vi "GOOP_WirePenTranslator.vi"(1 "WireConfigurationIn":T2, 3 "WirePensIn":T1(array[cluster])) -> (15 "WirePensOut":T1(array[cluster]), 17 "WireConfigurationOut":T2)   [LabVIEW 2020]
uses:
  <resource>/Framework/Providers/Open_GDS/SubVIs/GOOP_WireConfigurationType.ctl
  <resource>/Framework/Providers/Open_GDS/SubVIs/GOOP_WirePattern.ctl
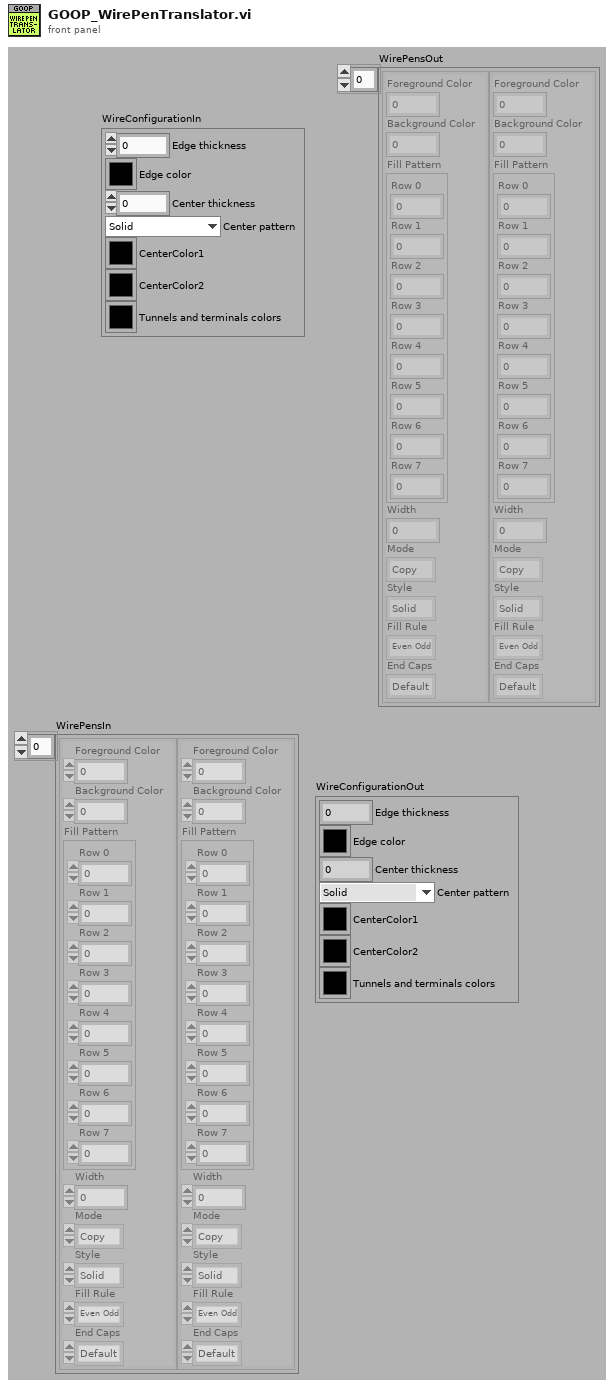
[diagram p1: front panel]
types:
  T1 = cluster{"Foreground Color":u32, "Background Color":u32, "Fill Pattern":cluster{"Row 0":u8, "Row 1":u8, "Row 2":u8, "Row 3":u8, "Row 4":u8, "Row 5":u8, "Row 6":u8, "Row 7":u8}, "Width":i16, "Mode":enum16{"Copy", "Or", "Exclusive Or", "Bit Clear", "Not Copy", "Not Or", "Nor Exclusive Or", "Not Bit Clear"}, "Style":enum32{"Solid", "Dash", "Dot", "Dash Dot", "Dash Dot Dot"}, "Fill Rule":enum32{"Even Odd", "Winding"}, "End Caps":enum32{"Default", "Flat"}}[]
  T2 = typedef "GOOP_WireConfigurationType.ctl" = cluster{"Edge thickness":i32, "Edge color":u32, "Center thickness":i32, "Center pattern":T3, "CenterColor1":u32, "CenterColor2":u32, "Tunnels and terminals colors":u32}
  T3 = typedef "GOOP_WirePattern.ctl" = enum16{"Solid", "Large dash", "Small dash"}
  T4 = cluster{"Row 0":u8, "Row 1":u8, "Row 2":u8, "Row 3":u8, "Row 4":u8, "Row 5":u8, "Row 6":u8, "Row 7":u8}
  T5 = cluster{"Foreground Color":u32, "Background Color":u32, "Fill Pattern":cluster{"Row 0":u8, "Row 1":u8, "Row 2":u8, "Row 3":u8, "Row 4":u8, "Row 5":u8, "Row 6":u8, "Row 7":u8}, "Width":i16, "Mode":enum16{"Copy", "Or", "Exclusive Or", "Bit Clear", "Not Copy", "Not Or", "Nor Exclusive Or", "Not Bit Clear"}, "Style":enum32{"Solid", "Dash", "Dot", "Dash Dot", "Dash Dot Dot"}, "Fill Rule":enum32{"Even Odd", "Winding"}, "End Caps":enum32{"Default", "Flat"}}
  T6 = cluster{"[0]":u8, "[1]":u8, "[2]":u8, "[3]":u8, "[4]":u8, "[5]":u8, "[6]":u8, "[7]":u8}
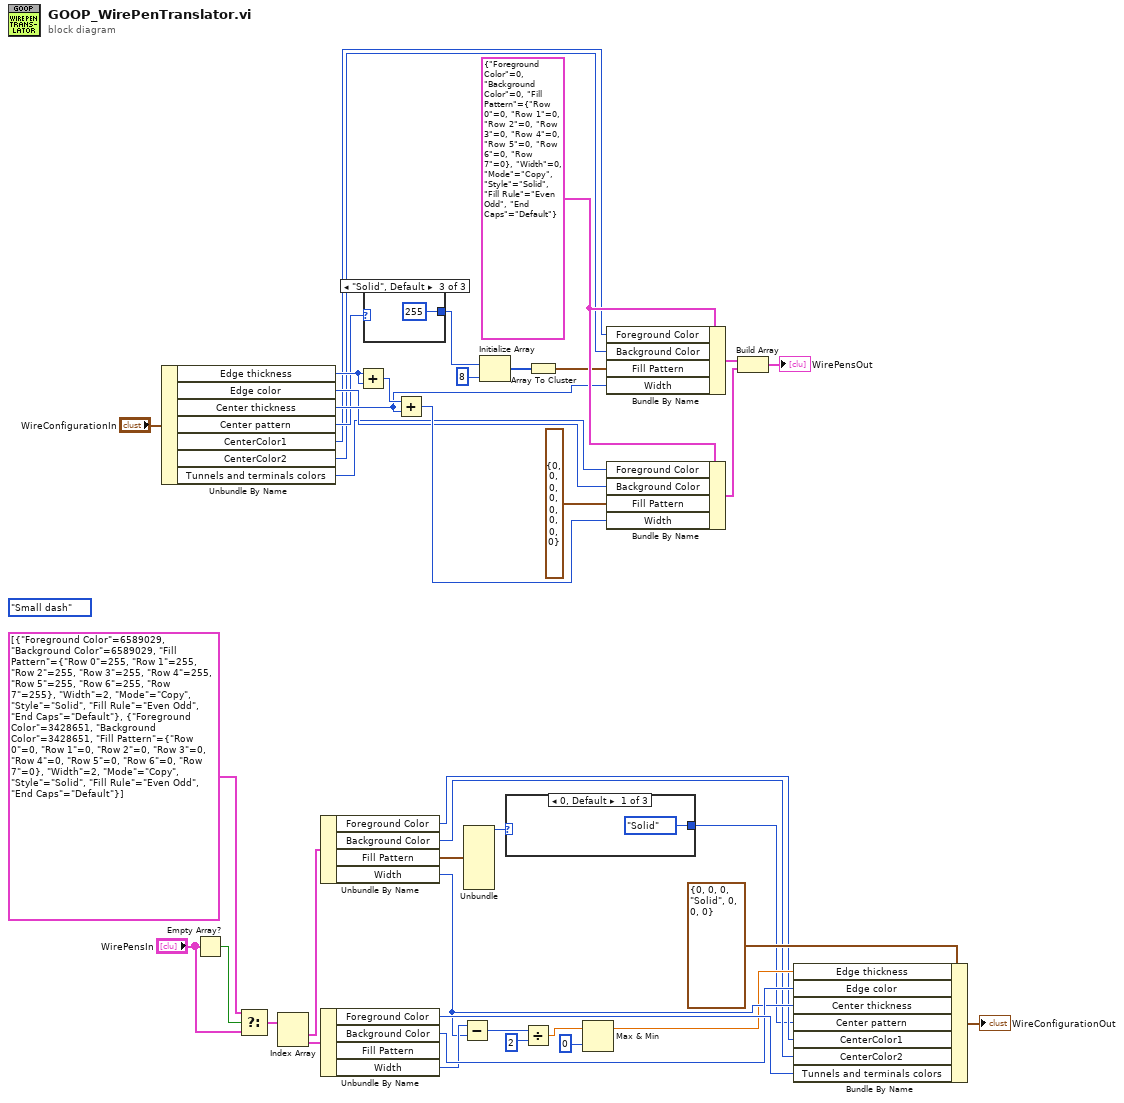
[diagram p0: block diagram]
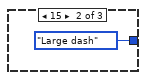
[diagram p2: hidden frame]
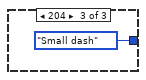
[diagram p3: hidden frame]
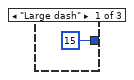
[diagram p4: hidden frame]
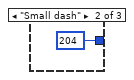
[diagram p5: hidden frame]
diagram:
  (unwired) GOOP_WirePattern."Small dash" ("Center pattern")
  w40 = T5 {"Foreground Color"=0, "Background Color"=0, "Fill Pattern"={"Row 0"=0, "Row 1"=0, "Row 2"=0, "Row 3"=0, "Row 4"=0, "Row 5"=0, "Row 6"=0, "Row 7"=0}, "Width"=0, "Mode"=enum."Copy", "Style"=enum."Solid", "Fill Rule"=enum."Even Odd", "End Caps"=enum."Default"} ("Pen")
  n1 = Unbundle By Name("WireConfigurationIn") -> ("Edge thickness"=w36:i32, "Edge color"=w32:u32, "Center thickness"=w34:i32, "Center pattern"=w31:T3, "CenterColor1"=w26:u32, "CenterColor2"=w25:u32, "Tunnels and terminals colors"=w24:u32)
  n2 = Empty Array?(array="WirePensIn") -> (empty?=w4:bool)
  n3 = Select(t=T1 [{"Foreground Color"=6589029, "Background Color"=6589029, "Fill Pattern"={"Row 0"=255, "Row 1"=255, "Row 2"=255, "Row 3"=255, "Row 4"=255, "Row 5"=255, "Row 6"=255, "Row 7"=255}, "Width"=2, "Mode"=enum."Copy", "Style"=enum."Solid", "Fill Rule"=enum."Even Odd", "End Caps"=enum."Default"}, {"Foreground Color"=3428651, "Background Color"=3428651, "Fill Pattern"={"Row 0"=0, "Row 1"=0, "Row 2"=0, "Row 3"=0, "Row 4"=0, "Row 5"=0, "Row 6"=0, "Row 7"=0}, "Width"=2, "Mode"=enum."Copy", "Style"=enum."Solid", "Fill Rule"=enum."Even Odd", "End Caps"=enum."Default"}] ("WirePensOut"), s=w4, f="WirePensIn") -> (s? t:f=w2:T1)
  n4 = Index Array(array=w2) -> (element #1=w22:T5, element #2=w21:T5)  [unwired: 2 in]
  n5 = Unbundle By Name(w22) -> ("Foreground Color"=w9:u32, "Background Color"=w8:u32, "Fill Pattern"=w7:T4, "Width"=w15:i16)
  n6 = Unbundle By Name(w21) -> ("Foreground Color"=w18:u32, "Background Color"=w17:u32, "Width"=w16:i16)  [unwired: 1 out]
  n7 = Add(x=w36, y=w36) -> (x+y=w35:i32)
  n8 = case shown="\"Solid\", Default" w31 {
    tunnel: [u8 15 ("Row 0") u8 204 ("Row 0") u8 255 ("Row 0")] -> w28
    frame "Large dash" {
    }
    frame "Small dash" {
    }
    frame "Solid", Default {
    }
  }
  n9 = Add(x=w35, y=w34) -> (x+y=w33:i32)
  n10 = Subtract(x=w16, y=w15) -> (x-y=w14:i16)
  n11 = Unbundle(w7) -> ("Row 0"=w6:u8)  [unwired: 7 out]
  n12 = Initialize Array(w28, 8 ("dimension size")) -> (w29:u8[])
  n13 = case shown="0, Default" w6 {
    tunnel: [GOOP_WirePattern."Solid" ("Center pattern") GOOP_WirePattern."Large dash" ("Center pattern") GOOP_WirePattern."Small dash" ("Center pattern")] -> w5
    frame 0, Default {
    }
    frame 15 {
    }
    frame 204 {
    }
  }
  n14 = Divide(x=w14, y=i16 2) -> (x/y=w12:dbl)
  n15 = Array To Cluster(array=w29) -> (cluster=w27:T6)
  n16 = Max & Min(x=w12, y=i16 0) -> (max(x,y)=w10:dbl)  [unwired: 1 out]
  n17 = Bundle By Name(cluster=w40, "Foreground Color"=w26, "Background Color"=w25, "Fill Pattern"=w27, "Width"=w34) -> (w39:T5)
  n18 = Bundle By Name(cluster=w40, "Foreground Color"=w24, "Background Color"=w32, "Fill Pattern"=T4 {"Row 0"=0, "Row 1"=0, "Row 2"=0, "Row 3"=0, "Row 4"=0, "Row 5"=0, "Row 6"=0, "Row 7"=0}, "Width"=w33) -> (w38:T5)
  n19 = Build Array(w39, w38) -> (→"WirePensOut":T1)
  n20 = Bundle By Name(cluster=T2 {"Edge thickness"=0, "Edge color"=0, "Center thickness"=0, "Center pattern"=enum."Solid", "CenterColor1"=0, "CenterColor2"=0, "Tunnels and terminals colors"=0} ("WireConfigurationOut"), "Edge thickness"=w10, "Edge color"=w17, "Center thickness"=w15, "Center pattern"=w5, "CenterColor1"=w9, "CenterColor2"=w8, "Tunnels and terminals colors"=w18) -> (→"WireConfigurationOut":T2)
